vi "Create-Ethernet-II.vi"(8 "Payload (in)":u8[](array[numeric])=[0, 1, 8, 0, 6, 4, 0, 1, 0, 35, 38, 182, 175, 53, 192, 168, 1, 200, 0, 0, 0, 0, 0, 0, 192, 168, 1, 201, 0, 0, 0, 0, 0, 0, 0, 0, 0, 0, 0, 0, 0, 0, 0, 0, 0, 0] format="%02x", 9 "EtherType":u16=2054 format="%04x", 10 "Source MAC":u8[](array[numeric])=[0, 35, 38, 182, 175, 53] format="%02x", 11 "Destination MAC":u8[](array[numeric])=[255, 255, 255, 255, 255, 255] format="%02x") -> (3 "Ethernet Frame (out)":u8[](array[numeric]) format="%02x")   [LabVIEW 2017]
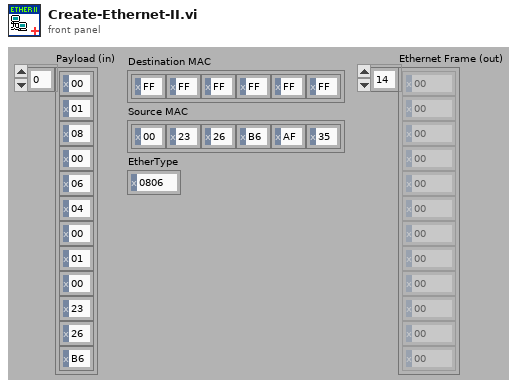
[diagram p1: front panel]
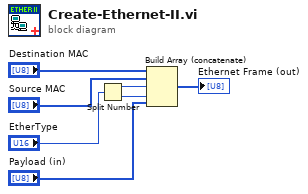
[diagram p0: block diagram]
diagram:
  n1 = Split Number(x="EtherType") -> (hi(x)=w3:u8, lo(x)=w2:u8)
  n2 = Build Array (concatenate)("Destination MAC", "Source MAC", w3, w2, "Payload (in)") -> (→"Ethernet Frame (out)":u8[])
